vi "Begin.vi"() -> (1 "Температура 2":string, 3 "Номер образца 2":string="538")   [LabVIEW 2018]
panel:
  in  "Температура":string="0"
  out "Boolean":bool=TRUE
  out "Ввел 2":bool=TRUE
  in  "Ввел":bool
  in  "Номер образца":string="0"
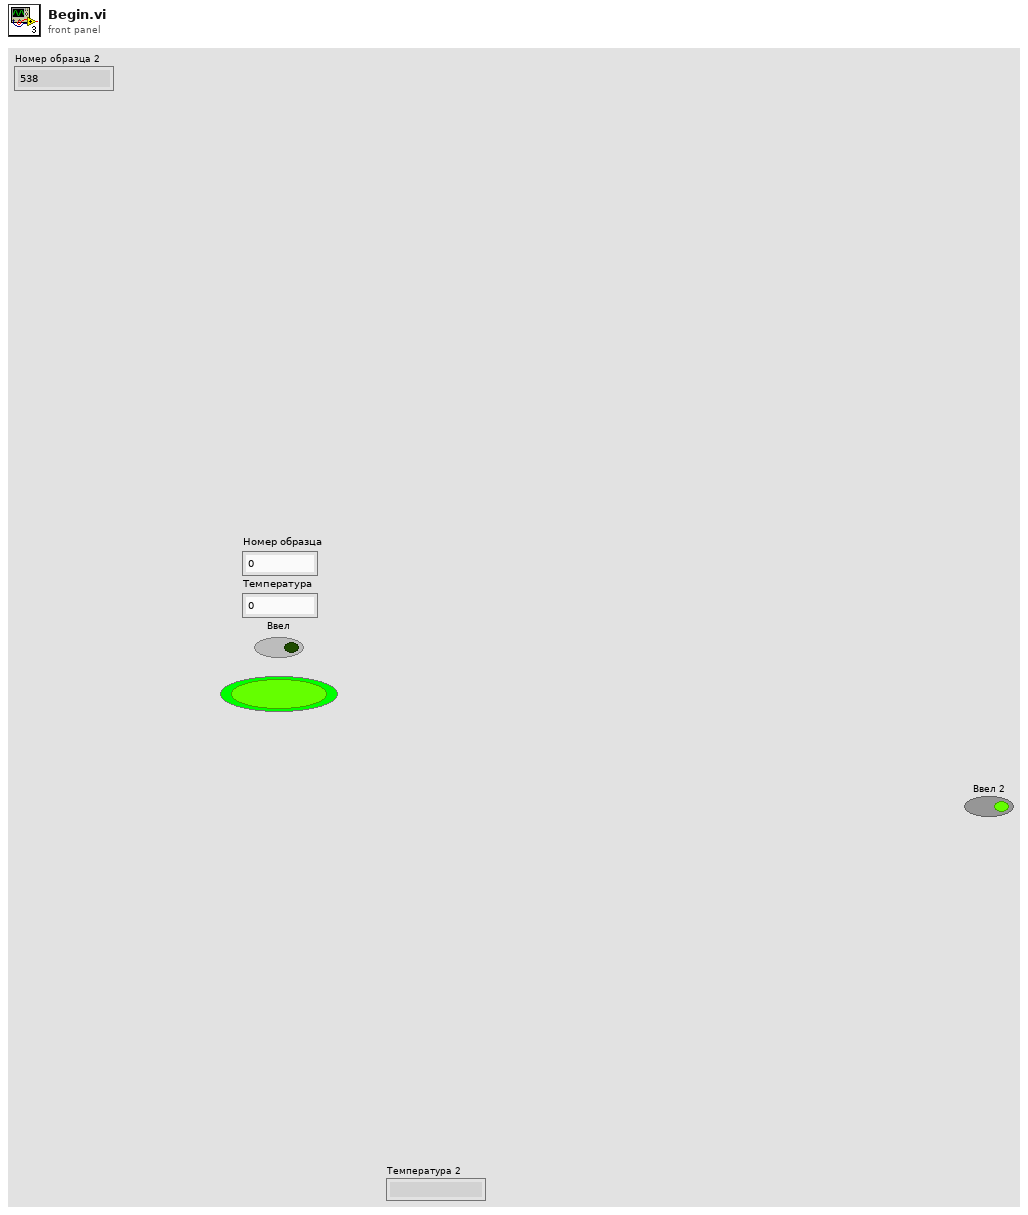
[diagram p1: front panel]
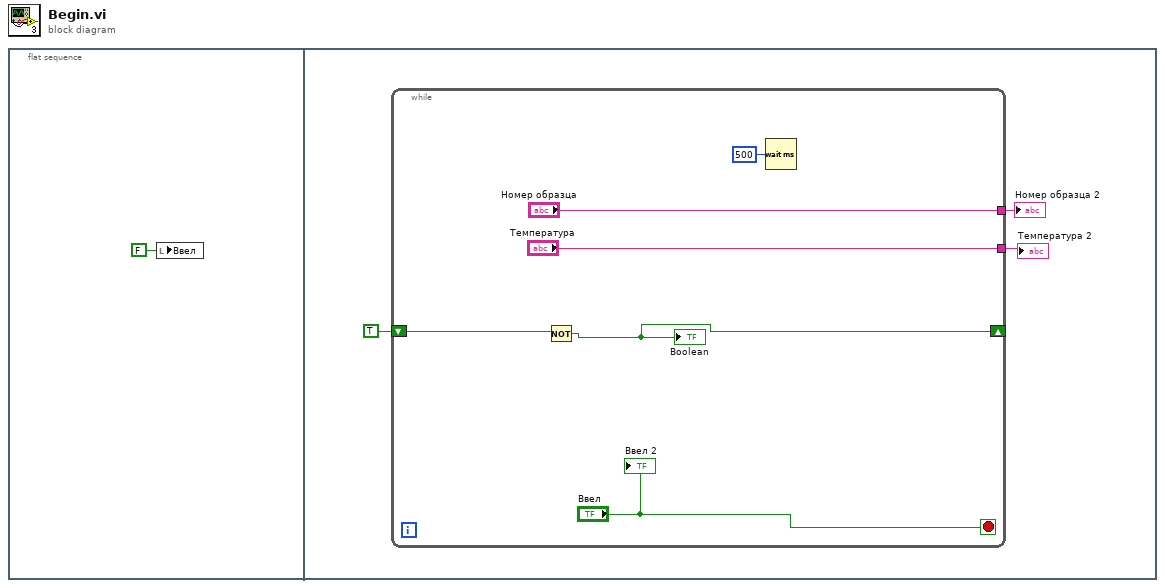
[diagram p0: block diagram]
diagram:
  n1 = flat-sequence {
    frame #0 {
      n2 = local write "Ввел"(FALSE ("Ввел")) -> ()
    }
    frame #1 {
      n3 = while {
        tunnel: ["Номер образца"] -> w4
        shift-right: [w6] -> _
        shift-left: TRUE -> [w7]
        tunnel: ["Температура"] -> w2
        stop <- "Ввел" stop-if-true
        n4 = Not(x=w7) -> (.not. x?=w6:bool)
        "Boolean" <- w6
        n5 = Wait (ms)(milliseconds to wait=u32 500) -> ()  [unwired: 1 out]
        "Ввел 2" <- "Ввел"
      }
      "Номер образца 2" <- w4
      "Температура 2" <- w2
    }
  }
